vi "save magnetometer readings.vi"(8 "error in":errorcluster, 10 "Magnetometer reading set":T1, 11 "input file":refnum<file>) -> (0 "error out":errorcluster, 3 "refnum out":refnum<file>)   [LabVIEW 2017]
uses:
  typedefs/magnetomter reading set.ctl
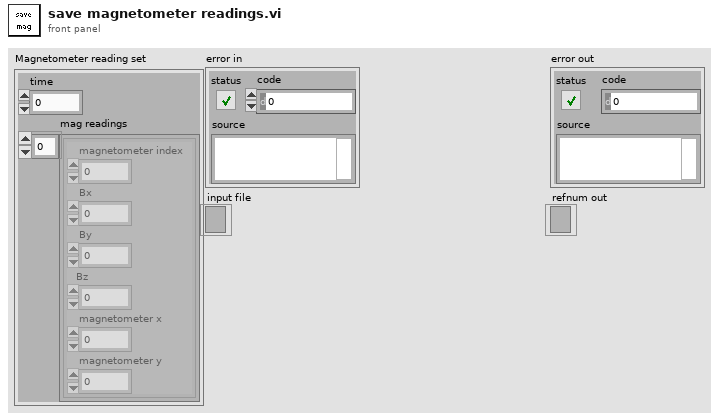
[diagram p1: front panel]
types:
  T1 = typedef "magnetomter reading set.ctl" = cluster{"time":fxp<+,48,48>, "mag readings":cluster{"magnetometer index":dbl, "Bx":dbl, "By":dbl, "Bz":dbl, "magnetometer x":dbl, "magnetometer y":dbl}[]}
  T2 = cluster{"magnetometer index":dbl, "Bx":dbl, "By":dbl, "Bz":dbl, "magnetometer x":dbl, "magnetometer y":dbl}[]
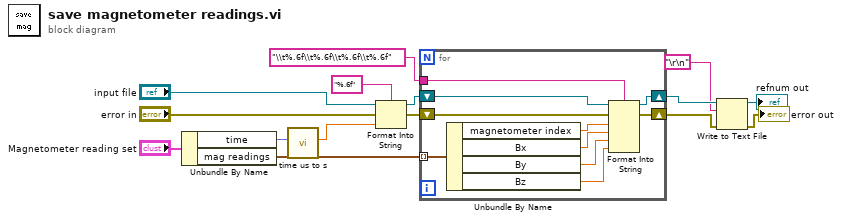
[diagram p0: block diagram]
diagram:
  n1 = Unbundle By Name("Magnetometer reading set") -> ("time"=w8:fxp<+,48,48>, "mag readings"=w13:T2)
  n2 = call "time us to s.vi"("time (us)"=w8) -> ("time (s)"=w7:dbl)  [unwired: 10 in]
  n3 = Format Into String(format string="%.6f", initial string="input file", error in="error in", w7) -> (resulting string=w10:refnum<file>, error out=w6:errorcluster)
  n4 = for {
    tunnel: "\\t%.6f\\t%.6f\\t%.6f\\t%.6f" ("format string") -> [w25]
    tunnel: w13 -> [w23] mode=indexing
    shift-right: [w17] -> w4
    shift-left: w6 -> [w22]
    shift-right: [w16] -> w5
    shift-left: w10 -> [w24]
    n5 = Unbundle By Name(w23) -> ("magnetometer index"=w18:dbl, "Bx"=w21:dbl, "By"=w20:dbl, "Bz"=w19:dbl)
    n6 = Format Into String(format string=w25, initial string=w24, error in=w22, w18, w21, w20, w19) -> (resulting string=w16:refnum<file>, error out=w17:errorcluster)
  }
  n7 = Write to Text File(file (use dialog)=w5, text="\r\n", error in=w4) -> (refnum out=→"refnum out":refnum<file>, error out=→"error out":errorcluster)  [unwired: 1 in, 1 out]
